vi "Setup RT Timetag.vi"(7 "Virtual Memory Unit in":refnum<class "Virtual Memory Unit.lvclass">, 8 "error in (no error)":errorcluster, 11 "Remote Terminal in":refnum<class "Remote Terminal.lvclass">) -> (0 "error out":errorcluster, 3 "Remote Terminal out":refnum<class "Remote Terminal.lvclass">, 5 "Virtual Memory Unit out":refnum<class "Virtual Memory Unit.lvclass">)   [LabVIEW 2020, in "BCI-1553 API.lvlib" / "Remote Terminal.lvclass"]
doc: "Setup the timetagging in use for the Remote Terminals.\n\nWe use a 2us internal clock tick for the internal timetagging. The holt chip is incapable of tagging value changes any faster than that. The internal timetags will change frequently and roll-over frequently with this configuration."
uses:
  Remote Terminal.lvclass
  Dependencies/Virtual Memory Unit/Virtual Memory Unit.lvclass
  Remote Terminal.lvclass/Remote Terminal.ctl
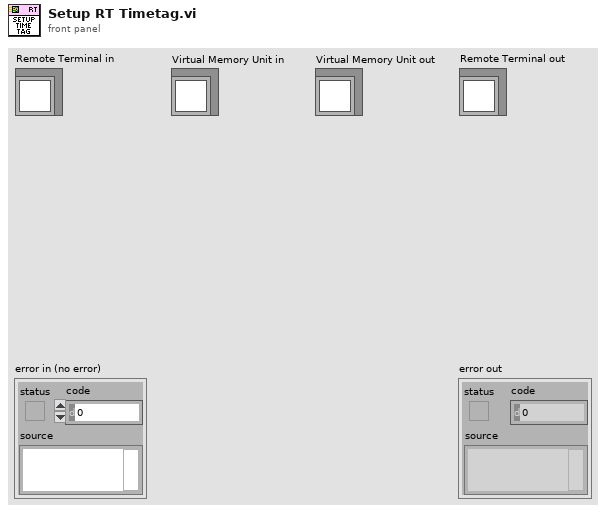
[diagram p1: front panel]
types:
  T1 = typedef "BCI-1553 API.lvlib/Remote Terminal.lvclass/RT Timetag Configuration.ctl" = enum16{"Disabled", "2us", "4us", "8us", "16us", "32us", "64us"}
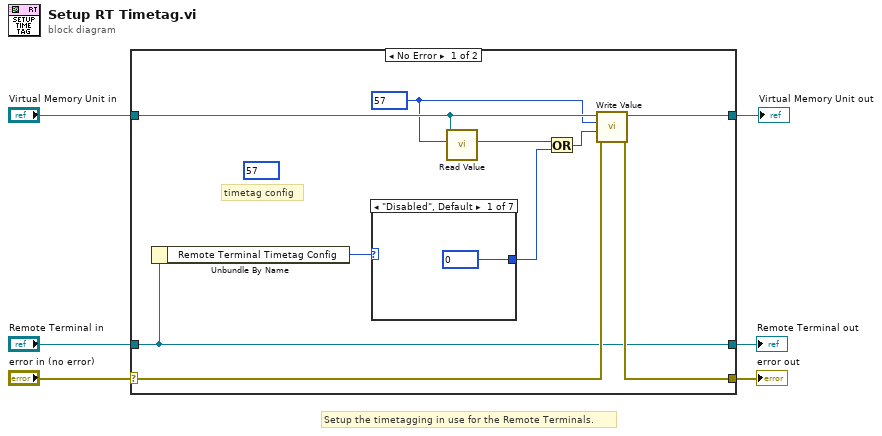
[diagram p0: block diagram]
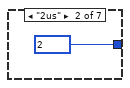
[diagram p2: hidden frame]
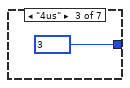
[diagram p3: hidden frame]
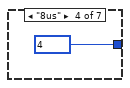
[diagram p4: hidden frame]
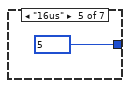
[diagram p5: hidden frame]
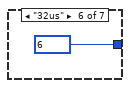
[diagram p6: hidden frame]
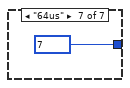
[diagram p7: hidden frame]
diagram:
  # "Setup the timetagging in use for the Remote Terminals."
  n1 = case shown="No Error" "error in (no error)" {
    selector: "error in (no error)" -> [w15 w26]
    tunnel: [w14 w26] -> w5
    tunnel: [w9 w25] -> w3
    tunnel: "Remote Terminal in" -> [w9 w25]
    tunnel: [w16 w24] -> w2
    tunnel: "Virtual Memory Unit in" -> [w13 w24]
    frame No Error {
      (unwired) u16 57 ("Address")
      w12 = 57 ("Address")
      # "timetag config"
      n2 = Unbundle By Name(w9) -> ("Remote Terminal Timetag Config"=w8:T1)
      n3 = case shown="\"Disabled\", Default" w8 {
        tunnel: [u16 0 ("Address") u16 2 ("Address") u16 3 ("Address") u16 4 ("Address") u16 5 ("Address") u16 6 ("Address") u16 7 ("Address")] -> w7
        frame "Disabled", Default {
        }
        frame "2us" {
        }
        frame "4us" {
        }
        frame "8us" {
        }
        frame "16us" {
        }
        frame "32us" {
        }
        frame "64us" {
        }
      }
      n4 = call "Read Value.vi"("Index"=w12, "Virtual Memory Unit in"=w13) -> ("Value"=w11:u16)  [unwired: 8 in, 1 out]
      n5 = Or(x=w11, y=w7) -> (x .or. y?=w10:u16)
      n6 = call "Write Value.vi"("error in (no error)"=w15, "Value"=w10, "Index"=w12, "Virtual Memory Unit in"=w13) -> ("error out"=w14:errorcluster, "Virtual Memory Unit out"=w16:refnum<class "Virtual Memory Unit.lvclass">)  [unwired: 6 in]
    }
    frame Error {
    }
  }
  "error out" <- w5
  "Remote Terminal out" <- w3
  "Virtual Memory Unit out" <- w2
